vi "R.vi"(9 "Q":dbl, 10 "L":dbl, 11 "f_rez":dbl) -> (3 "R":cdb)   [LabVIEW 2020]
doc: "SubVI wyznacza rezystancje na podstawie wartoœci dobroci.\n\nDane wejœciowe:\nf_rez - czêstotliwoœæ rezonansowa\nQ - dobroæ"
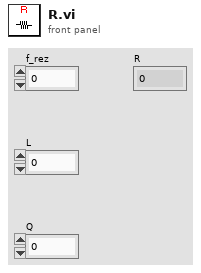
[diagram p1: front panel]
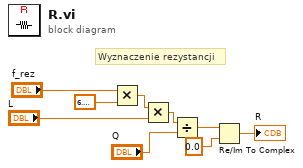
[diagram p0: block diagram]
diagram:
  # "Wyznaczenie rezystancji"
  n1 = Multiply(x="f_rez", y=6.283185307179586) -> (x*y=w4:dbl)
  n2 = Multiply(x=w4, y="L") -> (x*y=w5:dbl)
  n3 = Divide(x=w5, y="Q") -> (x/y=w7:dbl)
  n4 = Re/Im To Complex(1:0.0 ("y"), 2:w7) -> (0:→"R":cdb)
